vi "LeakyRelU Vector Elements.vi"(2 "X":T1, 6 "slope":dbl=0.01) -> (16 "RelU(X)":T1)   [LabVIEW 2014]
uses:
  <vilib>/Analysis/Matrix/Datatypes/RealMatrix.ctl
  <vilib>/Analysis/Matrix/NI_Matrix.lvlib
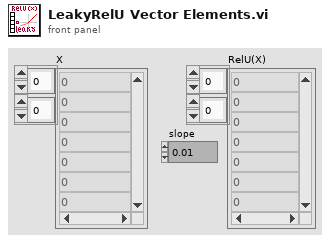
[diagram p1: front panel]
types:
  T1 = typedef "NI_Matrix.lvlib/RealMatrix.ctl" = dbl[][]
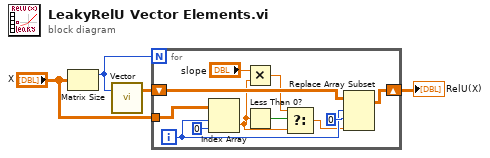
[diagram p0: block diagram]
diagram:
  n1 = Matrix Size(0:"X") -> (1:w3:i32)  [unwired: 1 out]
  n2 = call "Vector.vi"("length"=w3) -> ("Real Matrix (Column Vector)"=w2:T1)  [unwired: 18 in]
  n3 = for {
    N: w3 -> [_]
    tunnel: "X" -> [w12]
    shift-right: [w14] -> w1
    shift-left: w2 -> [w15]
    i -> [w11]
    n4 = Index Array(array=w12, index (row)=w11, index (col)=0) -> (element=w6:dbl)
    n5 = Multiply(x="slope", y=w6) -> (x*y=w5:dbl)
    n6 = Less Than 0?(x=w6) -> (x < 0?=w9:bool)
    n7 = Select(t=w5, s=w9, f=w6) -> (s? t:f=w8:dbl)
    n8 = Replace Array Subset(array=w15, new element=w8, index (row)=w11, index (col)=0 ("disabled index (col)")) -> (w14:T1)
  }
  "RelU(X)" <- w1
